vi "CALC_Normalize_1D_Array.vi"(2 "Error In":errorcluster, 4 "1D array":dbl[](array[numeric])) -> (0 "Error Out":errorcluster, 1 "Normalized 1D array":dbl[](array[numeric]))   [LabVIEW 2018, in "Tracker.lvlib"]
uses:
  Tracker.lvlib
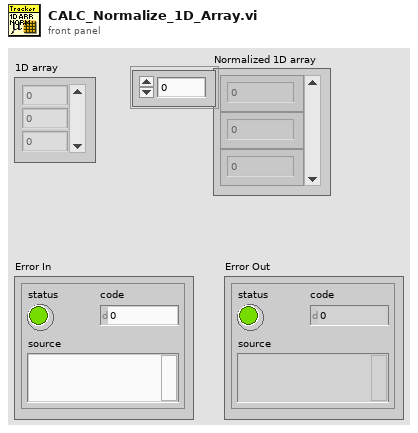
[diagram p1: front panel]
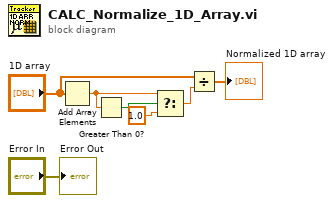
[diagram p0: block diagram]
diagram:
  n1 = Add Array Elements(numeric array="1D array") -> (sum=w2:dbl)
  n2 = Greater Than 0?(x=w2) -> (x > 0?=w6:bool)
  n3 = Select(t=w2, s=w6, f=1.0) -> (s? t:f=w5:dbl)
  n4 = Divide(x="1D array", y=w5) -> (x/y=→"Normalized 1D array":dbl[])
  "Error Out" <- "Error In"
